vi "EnergySystem.vi"() -> ()   [LabVIEW 2017]
uses:
  classes/DataCollector.lvclass
  classes/DataHandler.lvclass
  classes/SimulationParameter.lvclass
panel:
  out "Energy flow Inital":T1
  out "Day of Year":u32
  out "Energy flow External":T1
  out "Day Time":u32
  in  "Time Interval":u32=1
  in  "stop":bool
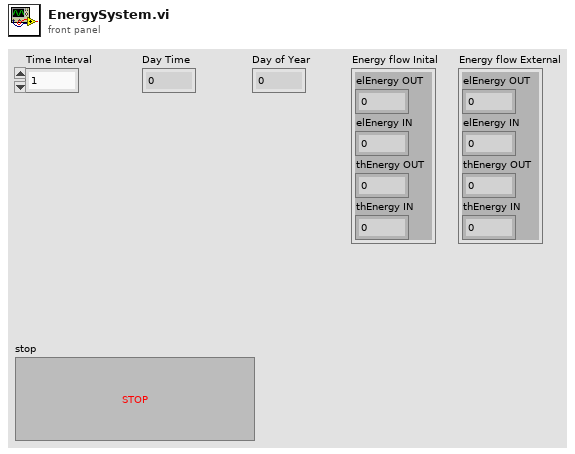
[diagram p1: front panel]
types:
  T1 = cluster{"elEnergy OUT":dbl, "elEnergy IN":dbl, "thEnergy OUT":dbl, "thEnergy IN":dbl}
  T2 = cluster{"DataCollector out":refnum<class "DataCollector.lvclass">, "DataHandler out":refnum<class "DataHandler.lvclass">, "SimulationParameter out":refnum<class "SimulationParameter.lvclass">}
  T3 = cluster{"DataCollector":refnum<class "DataCollector.lvclass">, "DataHandling":refnum<class "DataHandler.lvclass">, "SimulationParameter":refnum<class "SimulationParameter.lvclass">}
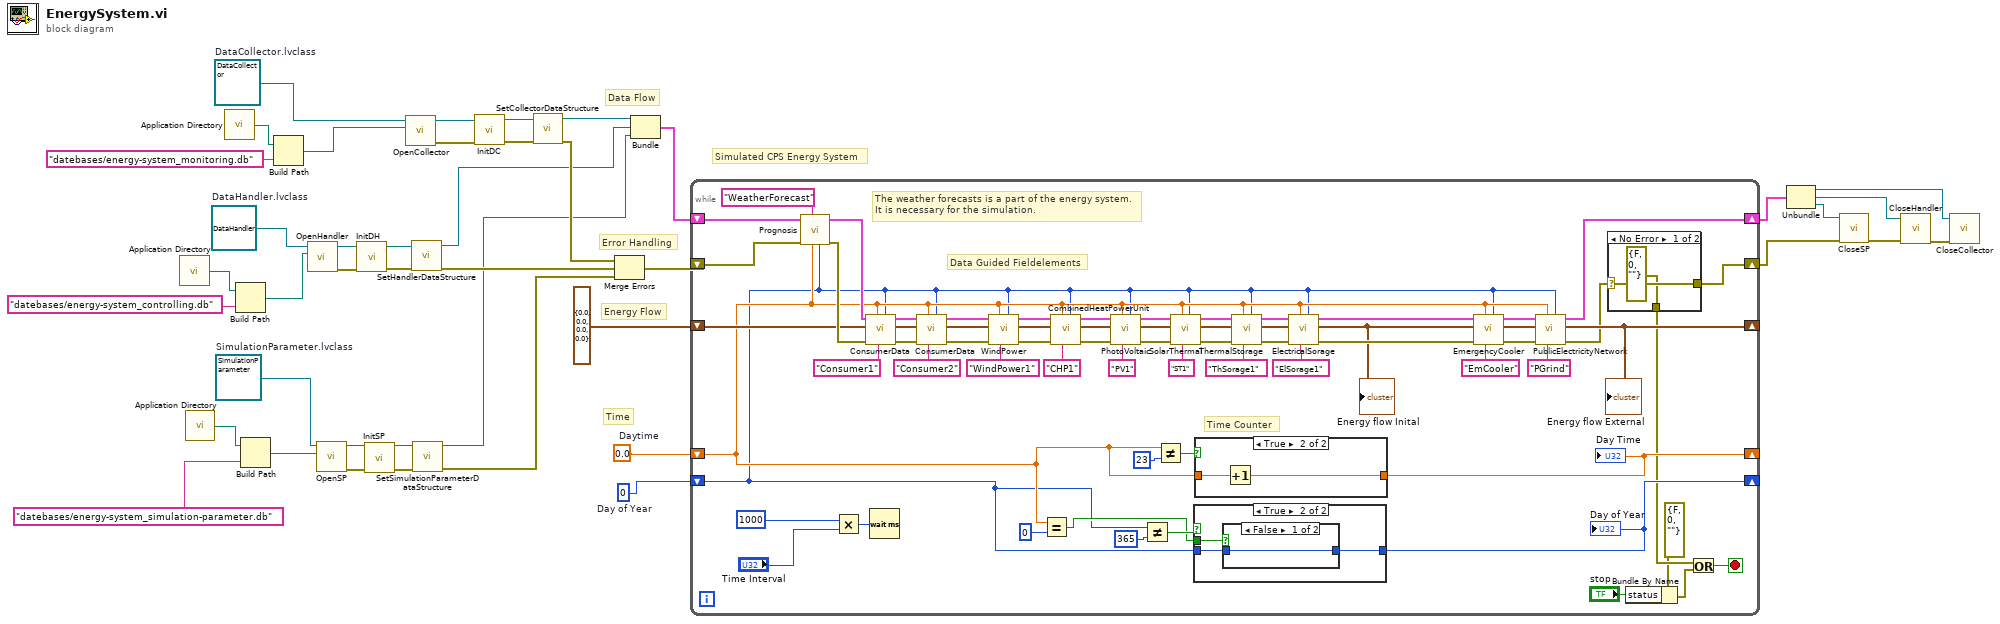
[diagram p0: block diagram]
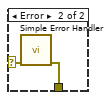
[diagram p2: hidden frame]
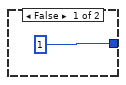
[diagram p3: hidden frame]
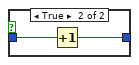
[diagram p4: hidden frame]
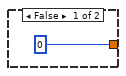
[diagram p5: hidden frame]
diagram:
  w8 = refnum<class "SimulationParameter.lvclass"> refnum  # SimulationParameter.lvclass
  w36 = refnum<class "DataHandler.lvclass"> refnum  # DataHandler.lvclass
  w35 = refnum<class "DataCollector.lvclass"> refnum  # DataCollector.lvclass
  w40 = u32 0  # Day of Year
  w41 = 0.0  # Daytime
  # "Error Handling"
  # "Simulated CPS Energy System"
  # "Data Flow"
  # "Time"
  # "Energy Flow"
  n1 = call <vilib>:"Application Directory.vi"() -> ("Application Directory"=w39:path)
  n2 = call <vilib>:"Application Directory.vi"() -> ("Application Directory"=w12:path)
  n3 = call <vilib>:"Application Directory.vi"() -> ("Application Directory"=w37:path)
  n4 = Build Path(base path=w39, name or relative path="datebases/energy-system_controlling.db" ("Name oder relativer Pfad")) -> (appended path=w38:path)
  n5 = Build Path(base path=w12, name or relative path="datebases/energy-system_simulation-parameter.db" ("Name oder relativer Pfad")) -> (appended path=w7:path)
  n6 = Build Path(base path=w37, name or relative path="datebases/energy-system_monitoring.db" ("Name oder relativer Pfad")) -> (appended path=w27:path)
  n7 = call-dynamic "OpenHandler.vi"("path to db monitoring"=w38, "DataHandling in"=w36) -> ("error out"=w21:errorcluster, "DataHandling out"=w20:refnum<class "DataHandler.lvclass">)  [unwired: 8 in]
  n8 = call-dynamic "OpenSP.vi"("path to db simulation"=w7, "SimulationParameter in"=w8) -> ("error out"=w5:errorcluster, "SimulationParameter out"=w6:refnum<class "SimulationParameter.lvclass">)  [unwired: 8 in]
  n9 = call-dynamic "InitDH.vi"("error in (no error)"=w21, "DataHandler in"=w20) -> ("error out"=w16:errorcluster, "DataHandler out"=w17:refnum<class "DataHandler.lvclass">)  [unwired: 8 in]
  n10 = call-dynamic "InitSP.vi"("error in (no error)"=w5, "SimulationParameter in"=w6) -> ("error out"=w4:errorcluster, "SimulationParameter out"=w3:refnum<class "SimulationParameter.lvclass">)  [unwired: 8 in]
  n11 = call-dynamic "OpenCollector.vi"("path to db monitoring"=w27, "DataCollector in"=w35) -> ("error out"=w22:errorcluster, "DataCollector out"=w25:refnum<class "DataCollector.lvclass">)  [unwired: 8 in]
  n12 = call-dynamic "SetHandlerDataStructure.vi"("error in (no error)"=w16, "DataHandler in"=w17) -> ("error out"=w14:errorcluster, "DataHandler out"=w15:refnum<class "DataHandler.lvclass">)  [unwired: 8 in]
  n13 = call-dynamic "SetSimulationParameterDataStructure.vi"("error in (no error)"=w4, "SimulationParameter in"=w3) -> ("error out"=w1:errorcluster, "SimulationParameter out"=w2:refnum<class "SimulationParameter.lvclass">)  [unwired: 8 in]
  n14 = call-dynamic "InitDC.vi"("error in (no error)"=w22, "DataCollector in"=w25) -> ("error out"=w23:errorcluster, "DataCollector out"=w24:refnum<class "DataCollector.lvclass">)  [unwired: 8 in]
  n15 = call-dynamic "SetCollectorDataStructure.vi"("error in (no error)"=w23, "DataCollector in"=w24) -> ("error out"=w18:errorcluster, "DataCollector out"=w26:refnum<class "DataCollector.lvclass">)  [unwired: 8 in]
  n16 = Merge Errors(w18, w14, w1) -> (w19:errorcluster)
  n17 = Bundle("DataCollector out"=w26, "DataHandler out"=w15, "SimulationParameter out"=w2) -> (w33:T2)  [unwired: 1 in]
  n18 = while {
    shift-right: [w84] -> _
    shift-left: T1 {"elEnergy OUT"=0.0, "elEnergy IN"=0.0, "thEnergy OUT"=0.0, "thEnergy IN"=0.0} ("Energy flow IN") -> [w53]
    shift-right: [w103] -> _
    shift-left: w41 -> [w46]
    shift-right: [w97] -> _
    shift-left: w40 -> [w45]
    shift-right: [w78] -> w10
    shift-left: w19 -> [w60]
    shift-right: [w83] -> w32
    shift-left: w33 -> [w61]
    stop <- w77 stop-if-true
    # "The weather forecasts is a part of the energy system.\nIt is necessary for the simulation."
    # "Data Guided Fieldelements"
    # "Time Counter"
    n19 = call "Prognosis.vi"("Day of Year"=w45, "Unique Object Identifier"="WeatherForecast", "Day Time"=w46, "Error In"=w60, "DataFlowIN"=w61) -> ("Error Out"=w57:errorcluster, "DataFlowOUT"=w52:T3)  [unwired: 5 in]
    n20 = Multiply(x=u32 1000, y="Time Interval") -> (x*y=w107:u32)
    n21 = call "ConsumerData.vi"("Day of Year"=w45, "Unique Object Identifier"="Consumer1", "Day Time"=w46, "Error In"=w57, "Energy flow IN"=w53, "DataFlowIN"=w52) -> ("Error Out"=w54:errorcluster, "Energy flow OUT"=w55:T1, "DataFlowOUT"=w56:T3)  [unwired: 3 in]
    n22 = Wait (ms)(milliseconds to wait=w107) -> ()  [unwired: 1 out]
    n23 = call "ConsumerData.vi"("Day of Year"=w45, "Unique Object Identifier"="Consumer2", "Day Time"=w46, "Error In"=w54, "Energy flow IN"=w55, "DataFlowIN"=w56) -> ("Error Out"=w62:errorcluster, "Energy flow OUT"=w63:T1, "DataFlowOUT"=w64:T3)  [unwired: 3 in]
    n24 = call "WindPower.vi"("Day of Year"=w45, "Unique Object Identifier"="WindPower1", "Day Time"=w46, "Error In"=w62, "Energy flow IN"=w63, "DataFlowIN"=w64) -> ("Error Out"=w82:errorcluster, "Energy flow OUT"=w81:T1, "DataFlowOUT"=w80:T3)  [unwired: 3 in]
    n25 = Equal?(x=w46, y=u32 0) -> (x = y?=w98:bool)
    n26 = call "CombinedHeatPowerUnit.vi"("Day of Year"=w45, "Unique Object Identifier"="CHP1", "Day Time"=w46, "Error In"=w82, "Energy flow IN"=w81, "DataFlowIN"=w80) -> ("Error Out"=w94:errorcluster, "Energy flow OUT"=w95:T1, "DataFlowOUT"=w96:T3)  [unwired: 3 in]
    n27 = call "PhotoVoltaic.vi"("Day of Year"=w45, "Unique Object Identifier"="PV1", "Day Time"=w46, "Error In"=w94, "Energy flow IN"=w95, "DataFlowIN"=w96) -> ("Error Out"=w93:errorcluster, "Energy flow OUT"=w92:T1, "DataFlowOUT"=w91:T3)  [unwired: 3 in]
    n28 = Not Equal?(x=w45, y=u32 365) -> (x != y?=w101:bool)
    n29 = Not Equal?(x=w46, y=u32 23) -> (x != y?=w100:bool)
    n30 = call "SolarThermal.vi"("Day of Year"=w45, "Unique Object Identifier"="ST1", "Day Time"=w46, "Error In"=w93, "Energy flow IN"=w92, "DataFlowIN"=w91) -> ("Error Out"=w89:errorcluster, "Energy flow OUT"=w87:T1, "DataFlowOUT"=w85:T3)  [unwired: 3 in]
    n31 = case shown="True" w101 {
      tunnel: [u32 1 ("Timer-Wert (ms)") w115] -> w97
      tunnel: w45 -> [_ w114]
      tunnel: w98 -> [_ w113]
      frame False {
      }
      frame True {
        n32 = case shown="False" w113 {
          tunnel: [w116 w118] -> w115
          tunnel: w114 -> [w116 w117]
          frame False {
          }
          frame True {
            n33 = Increment(x=w117) -> (x+1=w118:u32)
          }
        }
      }
    }
    "Day of Year" <- w97
    n34 = case shown="True" w100 {
      tunnel: [u32 0 ("Timer-Wert (ms)") w121] -> w103
      tunnel: w46 -> [_ w120]
      frame False {
      }
      frame True {
        n35 = Increment(x=w120) -> (x+1=w121:dbl)
      }
    }
    "Day Time" <- w103
    n36 = call "ThermalStorage.vi"("Day of Year"=w45, "Unique Object Identifier"="ThSorage1", "Day Time"=w46, "Error In"=w89, "Energy flow IN"=w87, "DataFlowIN"=w85) -> ("Error Out"=w90:errorcluster, "Energy flow OUT"=w88:T1, "DataFlowOUT"=w86:T3)  [unwired: 3 in]
    n37 = call "ElectricalSorage.vi"("Day of Year"=w45, "Unique Object Identifier"="ElSorage1", "Day Time"=w46, "Error In"=w90, "Energy flow IN"=w88, "DataFlowIN"=w86) -> ("Error Out"=w51:errorcluster, "Energy flow OUT"=w43:T1, "DataFlowOUT"=w48:T3)  [unwired: 3 in]
    "Energy flow Inital" <- w43
    n38 = call "EmergencyCooler.vi"("Day of Year"=w45, "Unique Object Identifier"="EmCooler", "Day Time"=w46, "Error In"=w51, "Energy flow IN"=w43, "DataFlowIN"=w48) -> ("Error Out"=w50:errorcluster, "Energy flow OUT"=w49:T1, "DataFlowOUT"=w47:T3)  [unwired: 3 in]
    n39 = call "PublicElectricityNetwork.vi"("Day of Year"=w45, "Unique Object Identifier"="PGrind", "Day Time"=w46, "Error In"=w50, "Energy flow IN"=w49, "DataFlowIN"=w47) -> ("Error Out"=w79:errorcluster, "Energy flow OUT"=w84:T1, "DataFlowOUT"=w83:T3)  [unwired: 3 in]
    "Energy flow External" <- w84
    n40 = case shown="No Error" w79 {
      selector: w79 -> [w109 w111]
      tunnel: [w109 _] -> w78
      tunnel: [errorcluster {"status"=FALSE, "code"=0, "source"=""} ("error out") w110] -> w76
      frame No Error {
      }
      frame Error {
        n41 = call <vilib>:"Simple Error Handler.vi"("error in (no error)"=w111) -> ("error out"=w110:errorcluster)  [unwired: 4 in, 4 out]
      }
    }
    n42 = Bundle By Name(cluster=errorcluster {"status"=FALSE, "code"=0, "source"=""} ("error out"), "status"="stop") -> (w73:errorcluster)
    n43 = Or(x=w76, y=w73) -> (x .or. y?=w77:bool)
  }
  n44 = Unbundle(w32) -> ("DataCollector out"=w31:refnum<class "DataCollector.lvclass">, "DataHandler out"=w30:refnum<class "DataHandler.lvclass">, "SimulationParameter out"=w11:refnum<class "SimulationParameter.lvclass">)
  n45 = call-dynamic "CloseSP.vi"("error in (no error)"=w10, "SimulationParameter in"=w11) -> ("error out"=w9:errorcluster)  [unwired: 8 in, 1 out]
  n46 = call-dynamic "CloseHandler.vi"("error in (no error)"=w9, "DataHandling in"=w30) -> ("error out"=w34:errorcluster)  [unwired: 8 in, 1 out]
  n47 = call "CloseCollector.vi"("error in (no error)"=w34, "DataCollector in"=w31) -> ()  [unwired: 8 in, 2 out]
